vi "Status.Update Error Cluster.vi"(6 "AddNewCode":bool, 7 "AppendOrigDesc":bool, 8 "Error In":errorcluster, 9 "NewDesc":string, 10 "NewCode":i32, 11 "Force Error":bool) -> (0 "Error Out":errorcluster)   [LabVIEW 2024, in "KATE_Lib.lvlib" / "Status Utils.lvlib"]
doc: "This VI will update the input error cluster information.\n\nIf Force Error = TRUE then the Error Out cluster will be set to:\n Status = True, Code = NewCode, Source = NewDesc\n\nIf Force Error = FALSE then\n The Error Out is only updated if the Error In Status is TRUE (contains an error)\n i.e. If there is no error input then the error out will also be no error.\n\nWhere Force Error = FALSE and Error In Status = TRUE \n If AppendOrigDesc = TRUE then\n The Error Out Source = NewDesc & \", \" & Error In Source \n Else\n The Error Out Source = NewDesc \n\n If NewCode is 0 then\n The Error Out Code = Error In Source \n Else if NewCode is not 0\n If AddCode = TRUE\n The Error Out Code = Error In Code + NewCode \n Else If AddCode = FALSE\n The Error Out Code = NewCode"
uses:
  Status Utils.lvlib
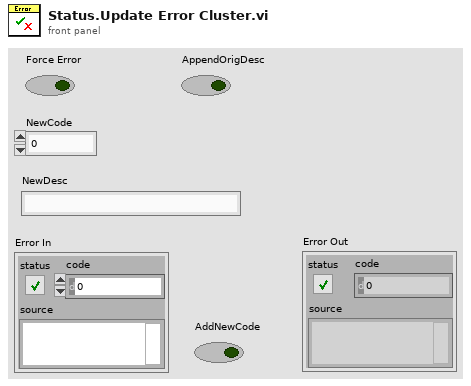
[diagram p1: front panel]
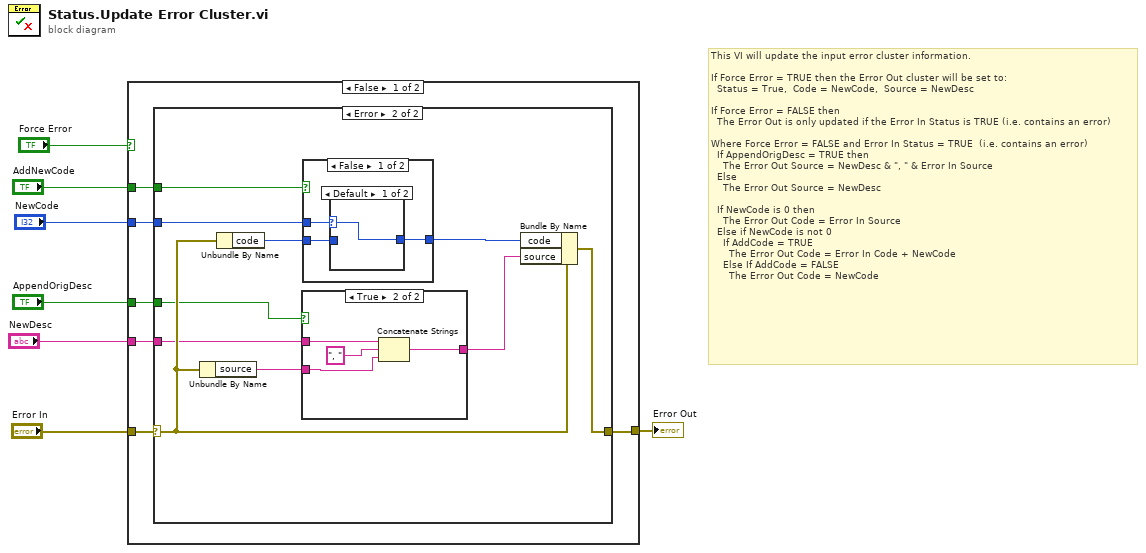
[diagram p0: block diagram]
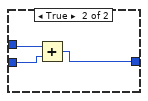
[diagram p6: hidden frame]
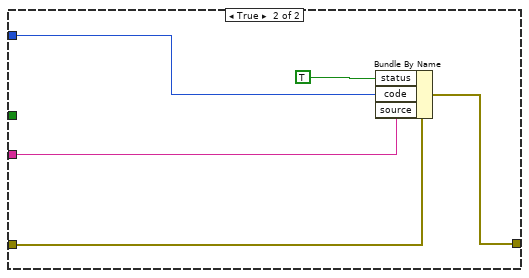
[diagram p7: hidden frame]
diagram:
  # "This VI will update the input error cluster information.\n\nIf Force Error = TRUE then the Error Out cluster will be set to:\n  Status = True,  Code = NewCode,  Source = NewDesc\n\nIf Force Error = FALSE then\n  The Error Out is only updated if the Error In Status is TRUE (i.e. contains an error)\n\nWhere Force Error = FALSE and Error In Status = TRUE  (i.e. contains an error) \n  If AppendOrigDesc = TRUE then\n    The Error Out Source = NewDesc & \", \" & Error In Source  \n  Else\n    The Error Out Source = NewDesc \n\n  If NewCode is 0 then\n    The Error Out Code = Error In Source  \n  Else if NewCode is not 0\n    If AddCode = TRUE\n      The Error Out Code = Error In Code + NewCode  \n    Else If AddCode = FALSE\n      The Error Out Code = NewCode"
  n1 = case shown="False" "Force Error" {
    tunnel: "NewCode" -> [w11 w44]
    tunnel: "NewDesc" -> [w10 w43]
    tunnel: "Error In" -> [w13 w46]
    tunnel: [w12 w45] -> w3
    tunnel: "AddNewCode" -> [w9 _]
    tunnel: "AppendOrigDesc" -> [w8 _]
    frame False {
      n2 = case shown="Error" w13 {
        selector: w13 -> [w14 w19]
        tunnel: [w14 w20] -> w12
        tunnel: w11 -> [_ w22]
        tunnel: w10 -> [_ w17]
        tunnel: w9 -> [_ w24]
        tunnel: w8 -> [_ w18]
        frame No Error {
        }
        frame Error {
          n3 = Unbundle By Name(w19) -> ("source"=w16:string)
          n4 = Unbundle By Name(w19) -> ("code"=w23:i32)
          n5 = case shown="True" w18 {
            tunnel: w17 -> [w27 w33]
            tunnel: w16 -> [w25 w31]
            tunnel: [w26 w30] -> w15
            frame False {
              n6 = case shown="Default" w27 {
                selector: w27 -> [w28 _]
                tunnel: [w28 w29] -> w26
                tunnel: w25 -> [_ w29]
                frame Default {
                }
                frame "" {
                }
              }
            }
            frame True {
              n7 = Concatenate Strings(w33, ", ", w31) -> (w30:string)
            }
          }
          n8 = case shown="False" w24 {
            tunnel: w23 -> [w34 w40]
            tunnel: w22 -> [w36 w41]
            tunnel: [w35 w39] -> w21
            frame False {
              n9 = case shown="Default" w36 {
                selector: w36 -> [w37 _]
                tunnel: [w37 w38] -> w35
                tunnel: w34 -> [_ w38]
                frame Default {
                }
                frame 0 {
                }
              }
            }
            frame True {
              n10 = Add(x=w41, y=w40) -> (x+y=w39:i32)
            }
          }
          n11 = Bundle By Name(cluster=w19, "code"=w21, "source"=w15) -> (w20:errorcluster)
        }
      }
    }
    frame True {
      n12 = Bundle By Name(cluster=w46, "status"=TRUE, "code"=w44, "source"=w43) -> (w45:errorcluster)
    }
  }
  "Error Out" <- w3
